vi "Get_SN_Coords.vi"(8 "Output EPOCH":dbl, 11 "ScopeSim._Telescope":refnum<k7>) -> (0 "DEC(sec)":dbl, 3 "RA(sec)":dbl)   [LabVIEW 2011]
panel:
  out "DEC":dbl format="%<%H:%M:%S>t"
  out "RA":dbl format="%<%H:%M:%S%1u>t"
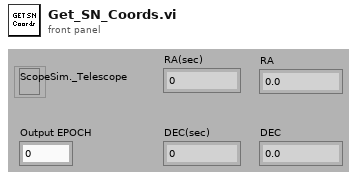
[diagram p1: front panel]
types:
  T1 = typedef "LVDateTimeRec.ctl" = cluster{"fractional second":dbl, "second":i32, "minute":i32, "hour":i32, "day of month":i32, "month":i32, "year":i32, "day of week":i32, "day of year":i32, "DST":i32}
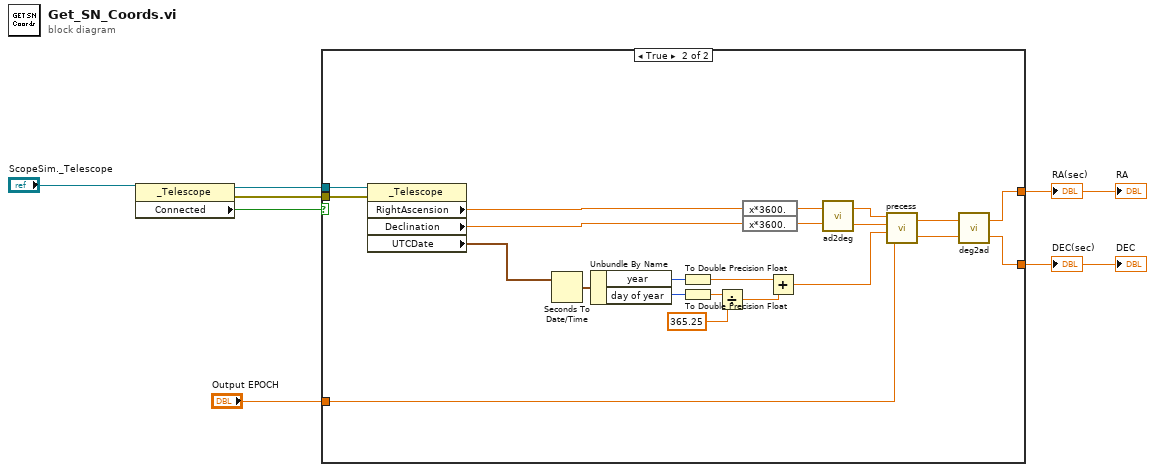
[diagram p0: block diagram]
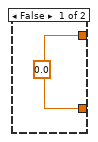
[diagram p2: hidden frame]
diagram:
  n1 = property class="_Telescope"(reference="ScopeSim._Telescope") -> (reference out=w7:refnum<k7>, error out=w6:errorcluster, "Connected"=w5:bool)  [unwired: 1 in]
  n2 = case shown="True" w5 {
    tunnel: w7 -> [_ w30]
    tunnel: w6 -> [_ w29]
    tunnel: [w8 w19] -> w3
    tunnel: [w8 w18] -> w2
    tunnel: "Output EPOCH" -> [_ w22]
    frame False {
      w8 = 0.0
    }
    frame True {
      n3 = property class="_Telescope"(reference=w30, error in=w29) -> ("RightAscension"=w28:dbl, "Declination"=w27:dbl, "UTCDate"=w17:timestamp)  [unwired: 2 out]
      n4 = Seconds To Date/Time(time stamp (now)=w17) -> (date time rec=w16:T1)  [unwired: 1 in]
      n5 = Unbundle By Name(w16) -> ("year"=w13:i32, "day of year"=w15:i32)
      n6 = To Double Precision Float(number=w13) -> (double precision float=w11:dbl)
      n7 = To Double Precision Float(number=w15) -> (double precision float=w14:dbl)
      n8 = Divide(x=w14, y=365.25) -> (x/y=w10:dbl)
      n9 = expression code="x*3600."(w28) -> (w26:dbl)
      n10 = expression code="x*3600."(w27) -> (w25:dbl)
      n11 = Add(x=w11, y=w10) -> (x+y=w9:dbl)
      n12 = call "ad2deg.vi"("DEC (sec)"=w25, "RA (sec)"=w26) -> ("DEC (°)"=w23:dbl, "RA (°)"=w24:dbl)
      n13 = call "precess.vi"("Eq2"=w22, "Eq1"=w9, "DEC 1"=w23, "RA 1"=w24) -> ("DEC 2"=w20:dbl, "RA 2"=w21:dbl)
      n14 = call "deg2ad.vi"("DEC (°)"=w20, "RA (°)"=w21) -> ("DEC (°)"=w18:dbl, "RA (sec)"=w19:dbl)
    }
  }
  "RA(sec)" <- w3
  "DEC(sec)" <- w2
  "RA" <- w3
  "DEC" <- w2
